vi "Set SessionOptions Ref.vi"(8 "error in (no error)":errorcluster, 10 "SessionOptions Ref":refnum<k24>, 11 "Session in":refnum<class "Session.lvclass">) -> (0 "error out":errorcluster, 3 "Session out":refnum<class "Session.lvclass">)   [LabVIEW 2015, in "WinSCP.lvlib" / "Session.lvclass"]
uses:
  Session.lvclass
  C:/Program Files (x86)/WinSCP/WinSCPnet.dll
  Program Files (x86)/WinSCP/WinSCPnet.dll
  Session.lvclass/Session.ctl
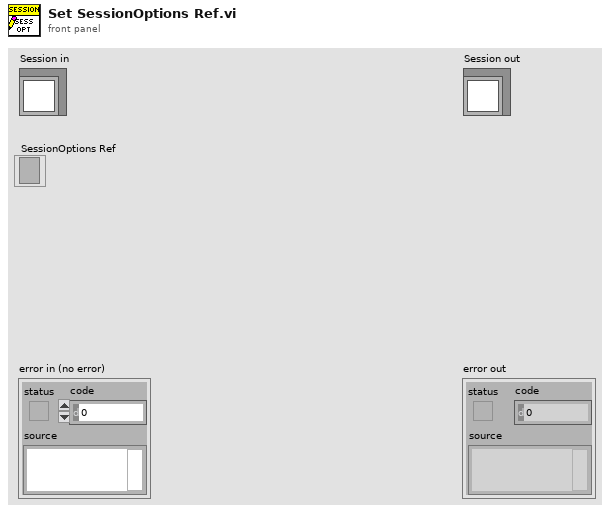
[diagram p1: front panel]
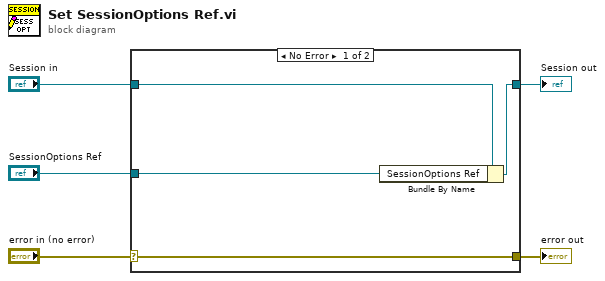
[diagram p0: block diagram]
diagram:
  n1 = case shown="No Error" "error in (no error)" {
    selector: "error in (no error)" -> [w9 w10]
    tunnel: [w9 w10] -> w4
    tunnel: [w7 w11] -> w2
    tunnel: "Session in" -> [w8 w11]
    tunnel: "SessionOptions Ref" -> [w6 _]
    frame No Error {
      n2 = Bundle By Name(cluster=w8, "SessionOptions Ref"=w6) -> (w7:refnum<class "Session.lvclass">)
    }
    frame Error {
    }
  }
  "error out" <- w4
  "Session out" <- w2
